vi "Test Error Propagation Lunit Verify CLI Output.vi"(8 "error in":errorcluster, 11 "Error.Tests in":refnum<class "Error.Propagation.Tests.lvclass">) -> (0 "error out":errorcluster, 3 "Error.Tests out":refnum<class "Error.Propagation.Tests.lvclass">)   [LabVIEW 2020, in "Error.Propagation.Tests.lvclass"]
uses:
  Error.Propagation.Tests.lvclass
  Source/Approval Tests/Options/Options.lvclass
  Source/Approval Tests/Verify CLI Options.ctl
  <vilib>/Astemes/LUnit/Test Case.lvclass
  <vilib>/addons/_JKI Toolkits/Caraya/classes/Assert/Assert True.vi
  <vilib>/addons/_JKI Toolkits/Caraya/classes/Assert/Assert Equal Value and Type_Variant.vi
  <vilib>/addons/_JKI Toolkits/Caraya/classes/Test/Test.lvclass
  <vilib>/addons/_JKI Toolkits/Caraya/classes/Assert/Assert.lvclass
  Source/Extensions/LUnit.Extension/LUnit.Extension.lvlib
  Source/Approval Tests/Approval Tests.lvlib
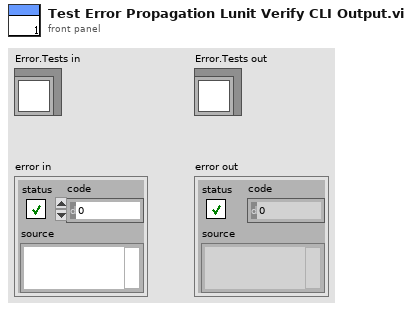
[diagram p1: front panel]
types:
  T1 = typedef "Approval Tests.lvlib/Verify CLI Options.ctl" = cluster{"standard input":string, "working directory":path, "expected output size  (4096)":u32, "Run Minimized (T)":bool}
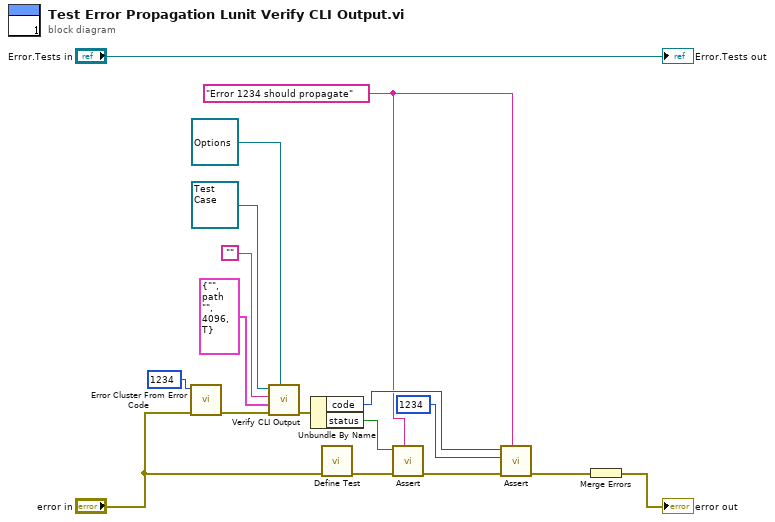
[diagram p0: block diagram]
diagram:
  w4 = "Error 1234 should propagate" ("Label (VI Title)")
  n1 = call <vilib>:"Error Cluster From Error Code.vi"("error in (no error)"="error in", "error code (0)"=1234) -> ("error out"=w14:errorcluster)  [unwired: 7 in]
  n2 = call "Verify CLI Output.vi"("Options"=refnum<class "Options.lvclass"> refnum, "error in"=w14, "CLI Options"=T1 {"standard input"="", "working directory"=path "", "expected output size  (4096)"=4096, "Run Minimized (T)"=TRUE}, "command line"="", "LUnit Test Case In"=refnum<class "Test Case.lvclass"> refnum) -> ("error out"=w13:errorcluster)  [unwired: 5 in, 1 out]
  n3 = Unbundle By Name(w13) -> ("code"=w6:i32, "status"=w7:bool)
  n4 = call <vilib>:"Define Test.vi"("error in (no error)"="error in") -> ("error out"=w17:errorcluster)  [unwired: 9 in, 1 out]
  n5 = call-poly <vilib>:"Assert.vi"("Label"=w4, "error in (no error)"=w17, "True?"=w7) -> ("error out"=w12:errorcluster)  [unwired: 7 in, 1 out]
  n6 = call-poly <vilib>:"Assert.vi"("Label"=w4, "error in (no error)"=w12, "Actual"=1234 ("error code (1)"), "Expected"=w6) -> ("error out"=w11:errorcluster)  [unwired: 6 in, 1 out]
  n7 = Merge Errors(w11) -> (→"error out":errorcluster)
  "Error.Tests out" <- "Error.Tests in"
